vi "DebTemplates.vi"(0 "Type":i32, 1 "Log":i32[](array[numeric]), 2 "Time":i32, 5 "error in":errorcluster) -> (19 "error out":errorcluster)   [LabVIEW 2017]
uses:
  DebCommandLog.vi
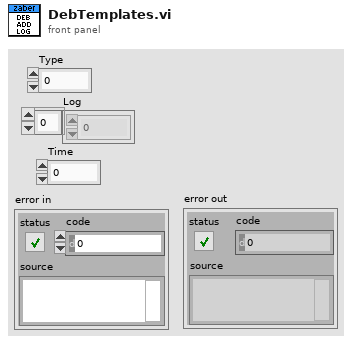
[diagram p1: front panel]
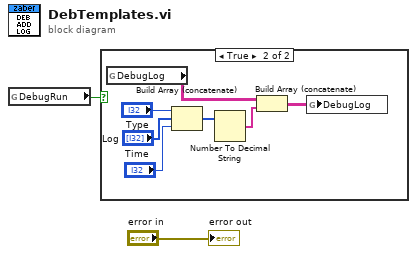
[diagram p0: block diagram]
diagram:
  n1 = global read "DebCommandLog.vi" "DebugRun"() -> (w1:bool)
  n2 = case shown="True" w1 {
    frame False {
    }
    frame True {
      n3 = global read "DebCommandLog.vi" "DebugLog"() -> (w9:string[][])
      n4 = Build Array (concatenate)("Type", "Log", "Time") -> (w4:i32[])
      n5 = Number To Decimal String(number=w4) -> (decimal integer string=w3:string[])  [unwired: 1 in]
      n6 = Build Array (concatenate)(w9, w3) -> (w8:string[][])
      n7 = global write "DebCommandLog.vi" "DebugLog"(w8) -> ()
    }
  }
  "error out" <- "error in"
